vi "RSNRPZ Read Buffer Data.vi"(7 "Channel (1)":i32=1, 8 "error in (no error)":errorcluster, 9 "Buffer Size (0)":i32, 10 "Maximum Time (5000 ms)":i32=5000, 11 "VISA session":refnum<visa-resource-name> caption="VISA resource name") -> (0 "error out":errorcluster, 1 "Read Count":i32, 2 "Measurement Array":dbl[](array[numeric]) format="%.3p", 3 "dup VISA session":refnum<visa-resource-name> caption="VISA resource name")   [LabVIEW 2010]
doc: "This VI initiates an acquisition on the channels that you specifies in channel parameter. It then waits for the acquisition to complete, and returns the measurement for the channel you specify."
uses:
  rsnrpz_32.dll
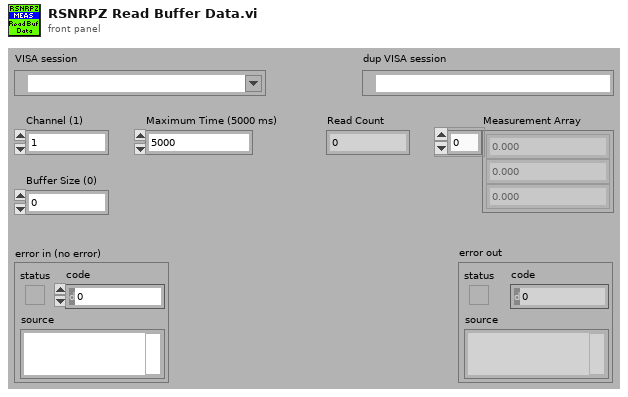
[diagram p1: front panel]
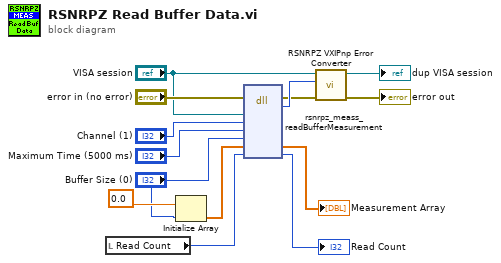
[diagram p0: block diagram]
diagram:
  n1 = local read "Read Count"() -> (w7:i32)
  n2 = Initialize Array(0.0, "Buffer Size (0)") -> (w9:dbl[])
  n3 = dll-call lib="rsnrpz_32.dll" fn="rsnrpz_meass_readBufferMeasurement"(error in="error in (no error)", "Instrument Handle"="VISA session", "Channel"="Channel (1)", "Maximum Time (ms)"="Maximum Time (5000 ms)", "Buffer Size"="Buffer Size (0)", w9, "Read Count"=w7) -> (error out=w5:errorcluster, "Status"=w13:i32, →"Measurement Array":dbl[], "Read Count"=→"Read Count":i32)  [unwired: 6 in, 1 out]
  n4 = call <instrlib>:"RSNRPZ VXIPnp Error Converter.vi"("error in"=w5, "VXIPnp error code"=w13, "VISA session"="VISA session") -> ("error out"=→"error out":errorcluster, "dup VISA session"=→"dup VISA session":refnum<visa-resource-name>)  [unwired: 7 in]
